vi "Configure Trigger (Runt).vi"(0 "VISA resource name":refnum<visa-resource-name>, 1 "Trigger Polarity (0: Positive)":u16(ring) items=["Positive", "Negative", "Either"], 5 "Trigger Source (0: Channel 1)":u16(ring) items=["Channel 1", "Channel 2", "Channel 3", "Channel 4", "RF"], 7 "High Threshold (0.8V)":dbl=0.8, 9 "Low Threshold (0.0V)":dbl, 11 "error in (no error)":errorcluster, 12 "Trigger Condition (0: Occurs)":u16(ring) items=["Occurs", "Less Than", "More Than", "Equal", "Not Equal"], 13 "Runt Width (4.0ns)":dbl=4e-09) -> (4 "VISA resource name out":refnum<visa-resource-name>, 15 "error out":errorcluster)   [LabVIEW 2017, in "Scope.lvlib" / "Tektronix DPO MSO 2000 4000 Series.lvlib"]
doc: "Configures runt trigger settings for an oscilloscope. A runt trigger occurs when the trigger signal crosses one of the runt thresholds twice without crossing the other runt threshold."
uses:
  Tektronix DPO MSO 2000 4000 Series.lvlib
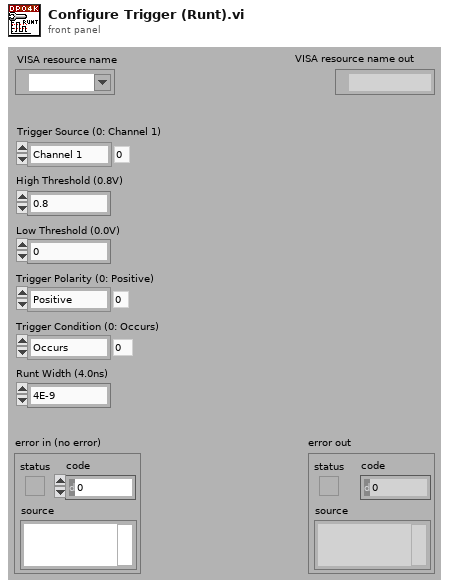
[diagram p1: front panel]
types:
  T1 = typedef "Scope.lvlib/Tektronix DPO MSO 2000 4000 Series.lvlib/Extended User Data.ctl" = cluster{"DPO MSO Series Model":u16}
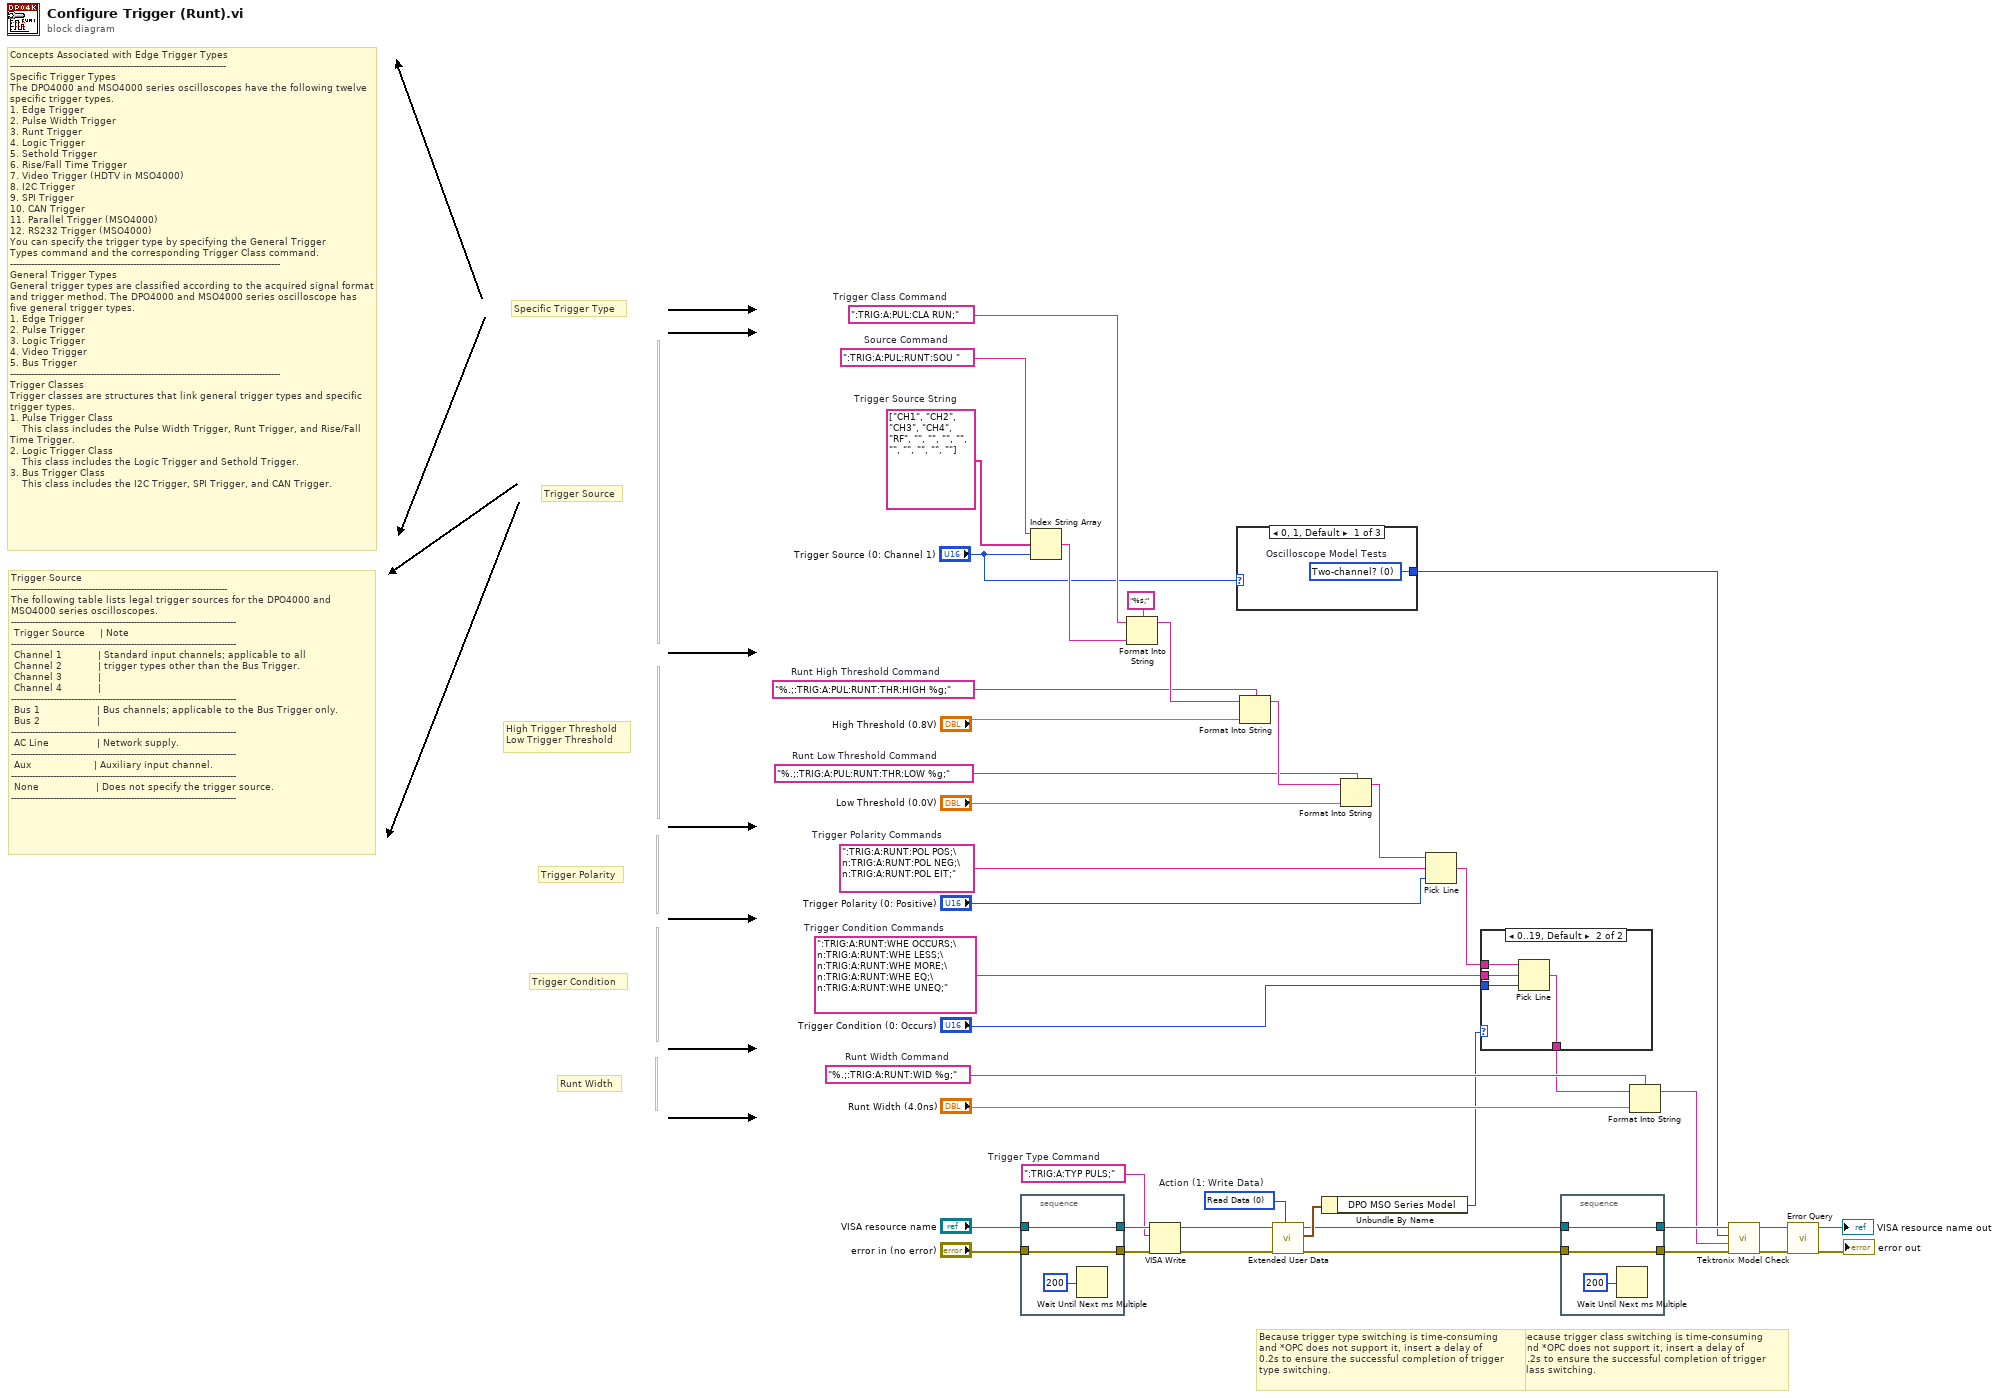
[diagram p0: block diagram]
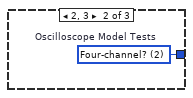
[diagram p2: hidden frame]
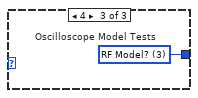
[diagram p3: hidden frame]
diagram:
  w6 = 0 items=["Read Data", "Write Data", "Clear Data", "Clear ALL Data"]  # Action (1: Write Data)
  w19 = string[] ["CH1", "CH2", "CH3", "CH4", "RF", "", "", "", "", "", "", "", "", ""]  # Trigger Source String
  w23 = "%.;:TRIG:A:RUNT:WID %g;"  # Runt Width Command
  w26 = ":TRIG:A:RUNT:WHE OCCURS;\n:TRIG:A:RUNT:WHE LESS;\n:TRIG:A:RUNT:WHE MORE;\n:TRIG:A:RUNT:WHE EQ;\n:TRIG:A:RUNT:WHE UNEQ;"  # Trigger Condition Commands
  w28 = ":TRIG:A:RUNT:POL POS;\n:TRIG:A:RUNT:POL NEG;\n:TRIG:A:RUNT:POL EIT;"  # Trigger Polarity Commands
  w30 = "%.;:TRIG:A:PUL:RUNT:THR:LOW %g;"  # Runt Low Threshold Command
  w32 = "%.;:TRIG:A:PUL:RUNT:THR:HIGH %g;"  # Runt High Threshold Command
  w38 = ":TRIG:A:PUL:RUNT:SOU "  # Source Command
  w36 = ":TRIG:A:PUL:CLA RUN;"  # Trigger Class Command
  w39 = ":TRIG:A:TYP PULS;"  # Trigger Type Command
  # "Trigger Source\n------------------------------------------------------------------------\nThe following table lists legal trigger sources for the DPO4000 and MSO4000 series oscilloscopes.\n---------------------------------------------------------------------------\n Trigger Source     | Note                                                           \n---------------------------------------------------------------------------\n Channel 1            | Standard input channels; applicable to all      \n Channel 2            | trigger types other than the Bus Trigger.         \n Channel 3            |     \n Channel 4            |\n---------------------------------------------------------------------------\n Bus 1                   | Bus channels; applicable to the Bus Trigger only.\n Bus 2                   | \n---------------------------------------------------------------------------\n AC Line                | Network supply.\n---------------------------------------------------------------------------\n Aux                     | Auxiliary input channel.\n---------------------------------------------------------------------------\n None                   | Does not specify the trigger source.\n---------------------------------------------------------------------------"
  # "Concepts Associated with Edge Trigger Types\n------------------------------------------------------------------------\nSpecific Trigger Types\nThe DPO4000 and MSO4000 series oscilloscopes have the following twelve specific trigger types.\n1. Edge Trigger\n2. Pulse Width Trigger\n3. Runt Trigger\n4. Logic Trigger\n5. Sethold Trigger\n6. Rise/Fall Time Trigger\n7. Video Trigger (HDTV in MSO4000)\n8. I2C Trigger\n9. SPI Trigger\n10. CAN Trigger\n11. Parallel Trigger (MSO4000)\n12. RS232 Trigger (MSO4000)\nYou can specify the trigger type by specifying the General Trigger \nTypes command and the corresponding Trigger Class command.\n------------------------------------------------------------------------------------------\nGeneral Trigger Types \nGeneral trigger types are classified according to the acquired signal format and trigger method. The DPO4000 and MSO4000 series oscilloscope has five general trigger types.\n1. Edge Trigger\n2. Pulse Trigger\n3. Logic Trigger\n4. Video Trigger\n5. Bus Trigger\n------------------------------------------------------------------------------------------\nTrigger Classes\nTrigger classes are structures that link general trigger types and specific trigger types.\n1. Pulse Trigger Class\n    This class includes the Pulse Width Trigger, Runt Trigger, and Rise/Fall Time Trigger.\n2. Logic Trigger Class\n    This class includes the Logic Trigger and Sethold Trigger.\n3. Bus Trigger Class\n    This class includes the I2C Trigger, SPI Trigger, and CAN Trigger."
  # "Because trigger class switching is time-consuming\nand *OPC does not support it, insert a delay of\n0.2s to ensure the successful completion of trigger\nclass switching."
  # "Because trigger type switching is time-consuming\nand *OPC does not support it, insert a delay of\n0.2s to ensure the successful completion of trigger\ntype switching."
  # "Runt Width"
  # "Trigger Condition"
  # "Trigger Polarity"
  # "High Trigger Threshold\nLow Trigger Threshold"
  # "Trigger Source"
  # "Specific Trigger Type"
  n1 = stacked-sequence {
    tunnel: "VISA resource name" -> [w43]
    tunnel: [w43] -> w41
    tunnel: "error in (no error)" -> [w42]
    tunnel: [w42] -> w40
    frame #0 {
      n2 = Wait Until Next ms Multiple(millisecond multiple=u32 200) -> ()  [unwired: 1 out]
    }
  }
  n3 = Index String Array(1:"Trigger Source (0: Channel 1)", 2:w19, 3:w38) -> (0:w37:string)
  n4 = Format Into String(format string="%s;", initial string=w36, w37) -> (resulting string=w34:string)  [unwired: 1 in, 1 out]
  n5 = VISA Write(VISA resource name=w41, write buffer=w39, error in (no error)=w40) -> (VISA resource name out=w5:refnum<visa-resource-name>, error out=w4:errorcluster)  [unwired: 1 out]
  n6 = case shown="0, 1, Default" "Trigger Source (0: Channel 1)" {
    tunnel: [w45 w46 w47] -> w8
    frame 0, 1, Default {
      w45 = u16 0 items=["Two-channel?", "Digital Model?", "Four-channel?", "RF Model?"]  # Oscilloscope Model Tests
    }
    frame 2, 3 {
      w46 = u16 2 items=["Two-channel?", "Digital Model?", "Four-channel?", "RF Model?"]  # Oscilloscope Model Tests
    }
    frame 4 {
      w47 = u16 3 items=["Two-channel?", "Digital Model?", "Four-channel?", "RF Model?"]  # Oscilloscope Model Tests
    }
  }
  n7 = Format Into String(format string=w32, initial string=w34, "High Threshold (0.8V)") -> (resulting string=w31:string)  [unwired: 1 in, 1 out]
  n8 = call "Extended User Data.vi"("Action (1: Write Data)"=w6, "error in (no error)"=w4, "VISA resource name"=w5) -> ("error out"=w2:errorcluster, "User Data Out"=w7:T1, "VISA resource name out"=w3:refnum<visa-resource-name>)  [unwired: 6 in]
  n9 = Unbundle By Name(w7) -> ("DPO MSO Series Model"=w1:u16)
  n10 = Format Into String(format string=w30, initial string=w31, "Low Threshold (0.0V)") -> (resulting string=w18:string)  [unwired: 1 in, 1 out]
  n11 = Pick Line(string ("")=w18, multi-line string=w28, line index="Trigger Polarity (0: Positive)") -> (output string=w17:string)
  n12 = case shown="0..19, Default" w1 {
    tunnel: w26 -> [_ w52]
    tunnel: "Trigger Condition (0: Occurs)" -> [_ w51]
    tunnel: [w48 w50] -> w22
    tunnel: w17 -> [w48 w49]
    frame 20, 27 {
    }
    frame 0..19, Default {
      n13 = Pick Line(string ("")=w49, multi-line string=w52, line index=w51) -> (output string=w50:string)
    }
  }
  n14 = stacked-sequence {
    tunnel: w3 -> [w54]
    tunnel: [w54] -> w14
    tunnel: w2 -> [w53]
    tunnel: [w53] -> w13
    frame #0 {
      n15 = Wait Until Next ms Multiple(millisecond multiple=u32 200) -> ()  [unwired: 1 out]
    }
  }
  n16 = Format Into String(format string=w23, initial string=w22, "Runt Width (4.0ns)") -> (resulting string=w10:string)  [unwired: 1 in, 1 out]
  n17 = call "Tektronix Model Check.vi"("error in (no error)"=w13, "Command String"=w10, "Oscilloscope Model Tests (3: RF Model?)"=w8, "VISA resource name"=w14) -> ("error out"=w11:errorcluster, "VISA resource name out"=w12:refnum<visa-resource-name>)  [unwired: 6 in]
  n18 = call "Error Query.vi"("error in (no error)"=w11, "VISA resource name"=w12) -> ("error out"=→"error out":errorcluster, "VISA resource name out"=→"VISA resource name out":refnum<visa-resource-name>)  [unwired: 6 in, 2 out]
